vi "DAQ_tb.vi"() -> ()   [LabVIEW 2018]
uses:
  <vilib>/DAQmx/read.llb/DAQmx Read (Analog Wfm 1Chan NSamp).vi
  <vilib>/DAQmx/create/channels.llb/DAQmx Create Channel (AI-Voltage-Basic).vi
  <vilib>/DAQmx/configure/timing.llb/DAQmx Timing (Sample Clock).vi
  <vilib>/DAQmx/miscellaneous.llb/DAQmx Fill In Error Info.vi
  <resource>/objmgr/daqmx.rc
panel:
  out "Sample Rate":dbl
  out "Waveform Graph 2":waveform(dbl)(graph)
  in  "Sample Clock Source":tag="OnboardClock"
  out "error out":errorcluster
  out "Actual Sample Rate":dbl=1000.0 format="%0.2f"
  in  "Sample Mode":i32(ring)=10123 items=["Finite Samples"=10178, "Continuous Samples"=10123, "Hardware Timed Single Point"=12522]
  in  "Terminal Configuration":i32(ring)=-1 items=["default"=-1, "RSE"=10083, "NRSE"=10078, "Differential"=10106, "Pseudodifferential"=12529]
  in  "Voltage Max Value":dbl=5.0 caption="Max Value"
  in  "Voltage Min Value":dbl=-5.0 caption="Min Value"
  in  "Voltage Physical Channels":tag="Dev1/ai0" caption="Physical Channels"
  in  "stop":bool
  out "Waveform Graph":waveform(dbl)(graph)
  in  "Sample rate":enum16{"1KHz", "10KHz", "100KHz", "1MHz"}(ring)
  in  "Time":dbl
  out "N Samples":dbl
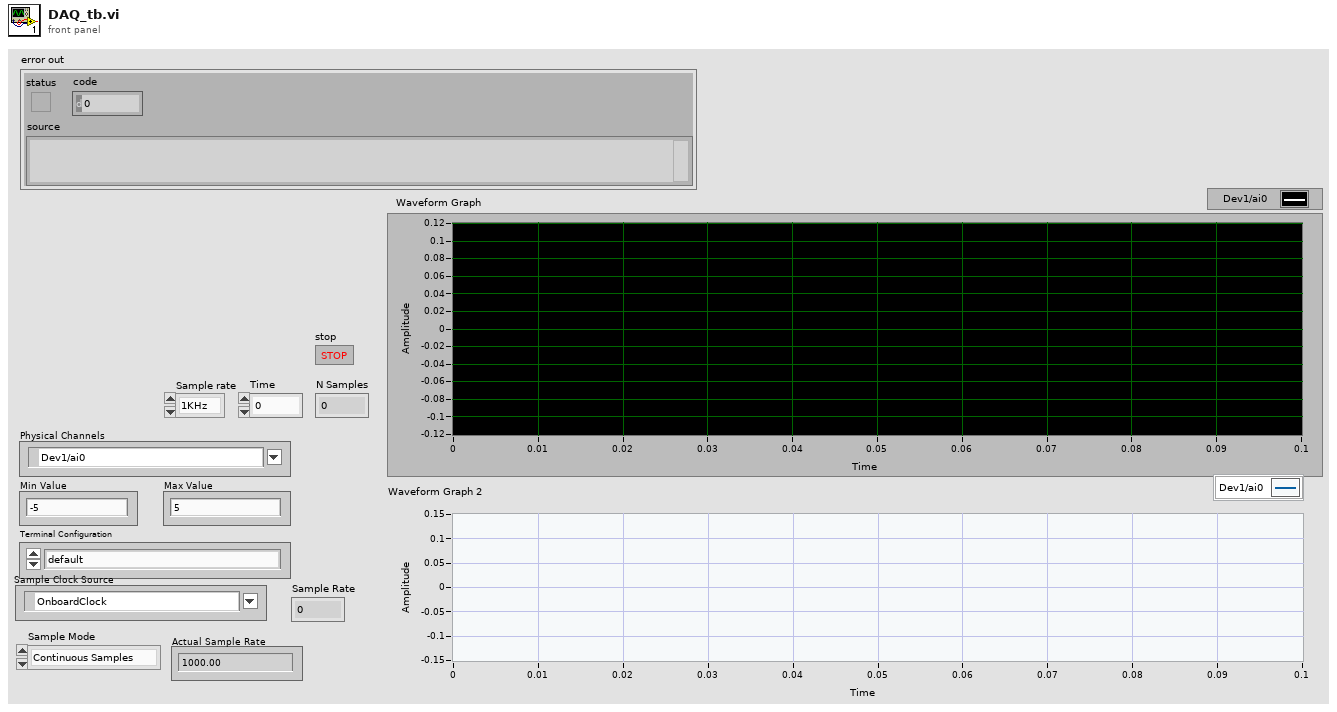
[diagram p1: front panel]
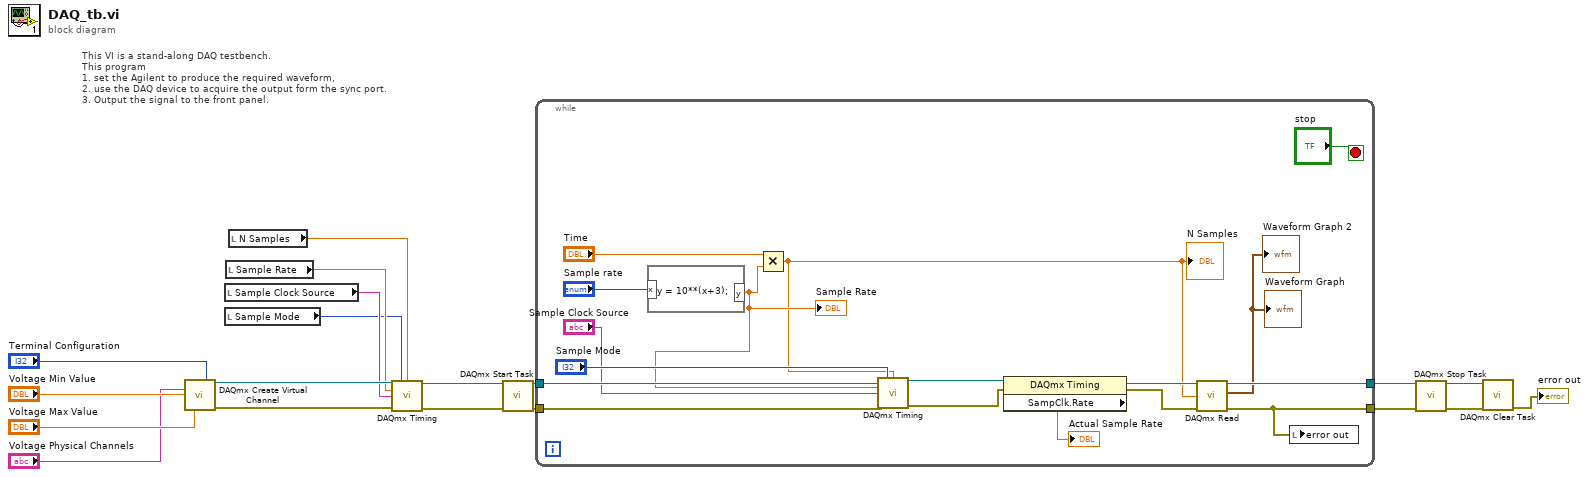
[diagram p0: block diagram]
diagram:
  # "This VI is a stand-along DAQ testbench.  \nThis program \n1. set the Agilent to produce the required waveform,\n2. use the DAQ device to acquire the output form the sync port. \n3. Output the signal to the front panel."
  n1 = call-poly <vilib>:"DAQmx Create Virtual Channel.vi"("maximum value"="Voltage Max Value", "minimum value"="Voltage Min Value", "input terminal configuration"="Terminal Configuration", "physical channels"="Voltage Physical Channels") -> ("task out"=w6:refnum<k21>, "error out"=w5:errorcluster)  [unwired: 10 in]
  n2 = local read "Sample Clock Source"() -> (w4:tag)
  n3 = local read "Sample Mode"() -> (w2:i32)
  n4 = local read "Sample Rate"() -> (w3:dbl)
  n5 = local read "N Samples"() -> (w1:dbl)
  n6 = call-poly <vilib>:"DAQmx Timing.vi"("task/channels in"=w6, "sample mode"=w2, "samples per channel"=w1, "rate"=w3, "source"=w4, "error in"=w5) -> ("task out"=w7:refnum<k21>, "error out"=w8:errorcluster)  [unwired: 8 in]
  n7 = call <vilib>:"DAQmx Start Task.vi"("task/channels in"=w7, "error in"=w8) -> ("task out"=w15:refnum<k21>, "error out"=w14:errorcluster)  [unwired: 12 in]
  n8 = while {
    tunnel: w15 -> [w31]
    tunnel: w14 -> [w30]
    tunnel: [w35] -> w13
    tunnel: [w21] -> w12
    stop <- "stop" stop-if-true
    n9 = formula code="y = 10**(x+3);"("x"="Sample rate") -> ("y"=w28:dbl)
    "Sample Rate" <- w28
    n10 = Multiply(x="Time", y=w28) -> (x*y=w20:dbl)
    "N Samples" <- w20
    n11 = call-poly <vilib>:"DAQmx Timing.vi"("task/channels in"=w31, "sample mode"="Sample Mode", "samples per channel"=w20, "rate"=w28, "source"="Sample Clock Source", "error in"=w30) -> ("task out"=w26:refnum<k21>, "error out"=w22:errorcluster)  [unwired: 8 in]
    n12 = property class="DAQmx Timing"(reference=w26, error in=w22) -> (reference out=w25:refnum<k21>, error out=w24:errorcluster, "SampClk.Rate"=→"Actual Sample Rate":dbl)
    n13 = call-poly <vilib>:"DAQmx Read.vi"("task/channels in"=w25, "number of samples per channel"=w20, "error in"=w24) -> ("task out"=w35:refnum<k21>, "data"=→"Waveform Graph" →"Waveform Graph 2":waveform(dbl), "error out"=w21:errorcluster)  [unwired: 10 in]
    n14 = local write "error out"(w21) -> ()
  }
  n15 = call <vilib>:"DAQmx Stop Task.vi"("task/channels in"=w13, "error in"=w12) -> ("task out"=w11:refnum<k21>, "error out"=w10:errorcluster)  [unwired: 12 in]
  n16 = call <vilib>:"DAQmx Clear Task.vi"("task in"=w11, "error in"=w10) -> ("error out"=→"error out":errorcluster)  [unwired: 13 in]
